vi "Subpanel.vi"() -> ()   [LabVIEW 2013]
panel:
  in  "Stop":bool
  in  "error in (no error)":errorcluster
  in  "RESET":bool
  in  "Feed Sel":bool
  in  "PCV Sel":bool
  in  "Boolean 10":bool
  in  "Boolean 9":bool
  in  "VLS Sel 1":bool
  in  "VLS Sel":bool
  in  "AKO Sel 2":bool
  in  "AKO Sel 1":bool
  in  "AKO Sel":bool
  in  "RX Sel":bool
  in  "MFC Sel":bool
  in  "Display Window":u16(ring) items=["Rx", "Guage", "PIDs", "Feed", "MFC", "AKO", "Steam", "Quench", "Back Half", "Heat Tapes"]
  in  "E-STOP":bool
  out "Estop":bool
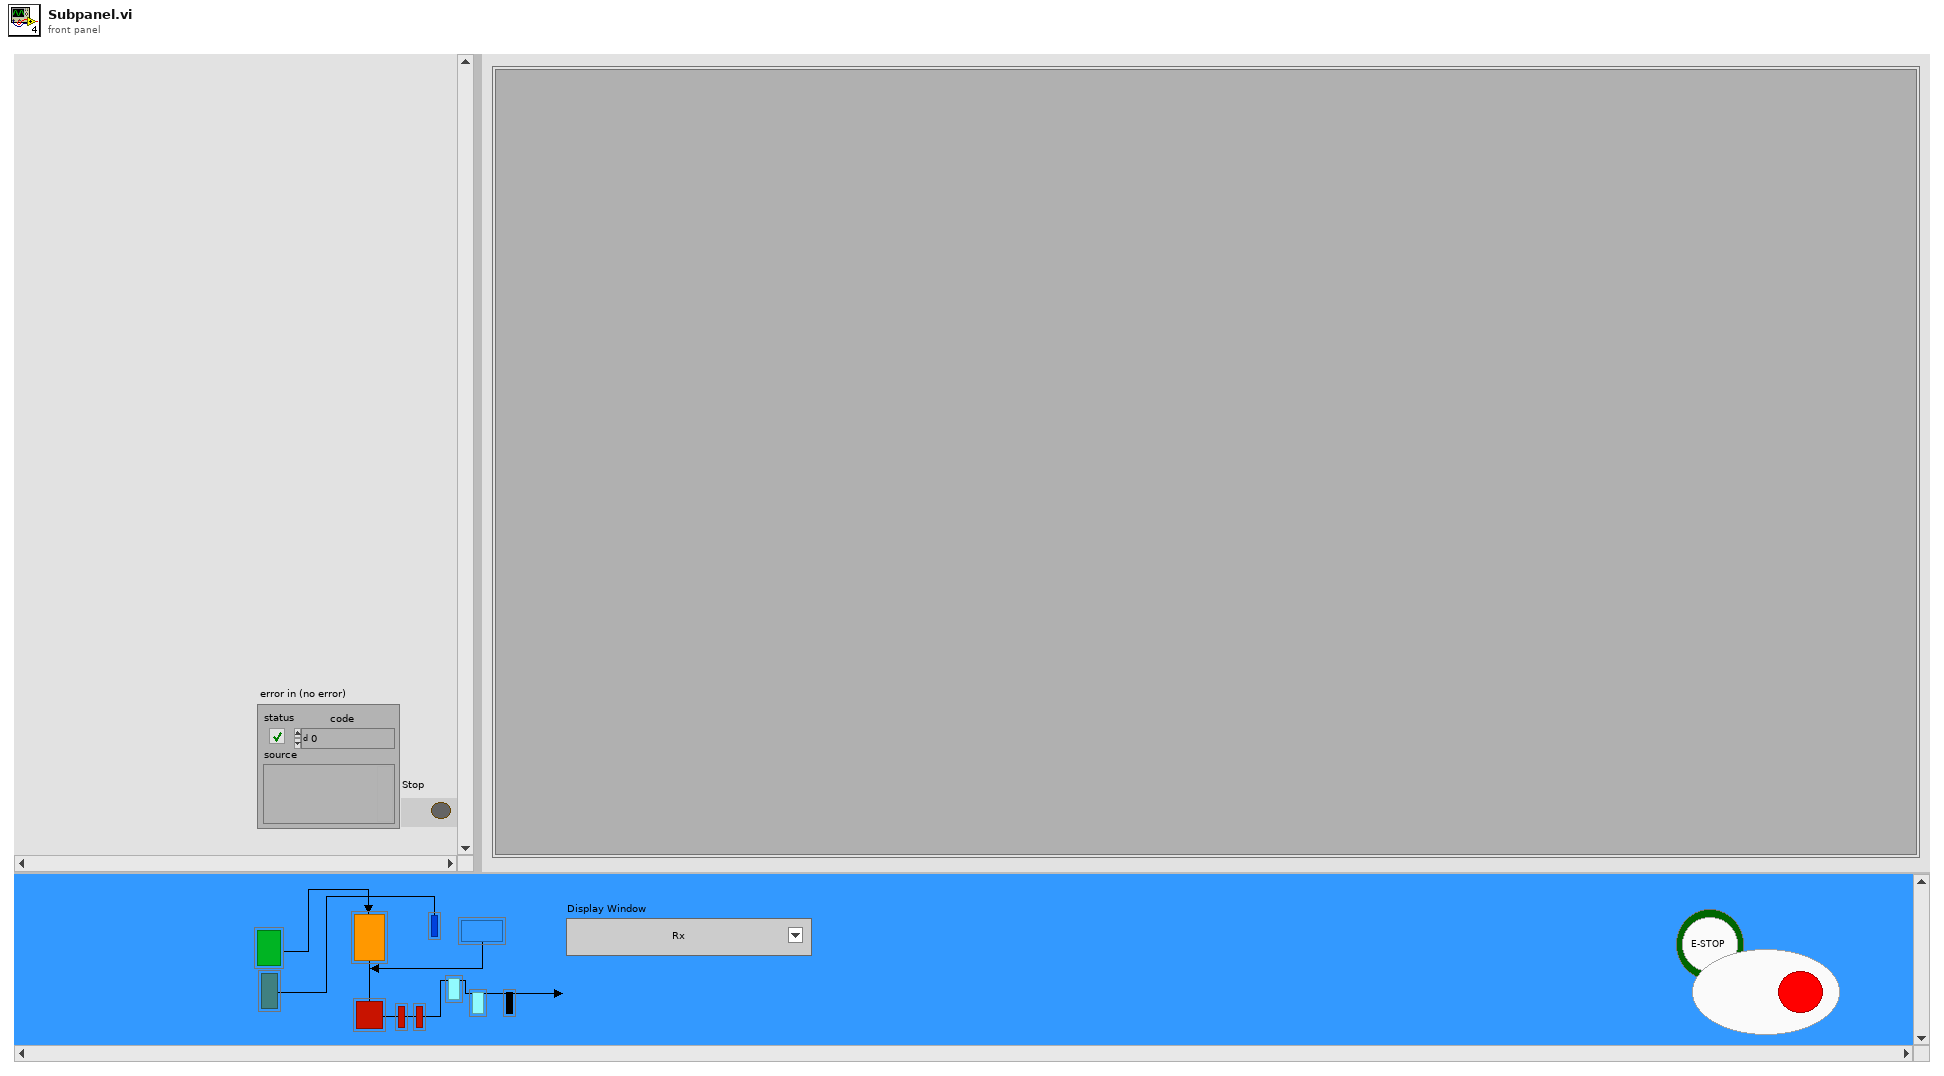
[diagram p1: front panel]
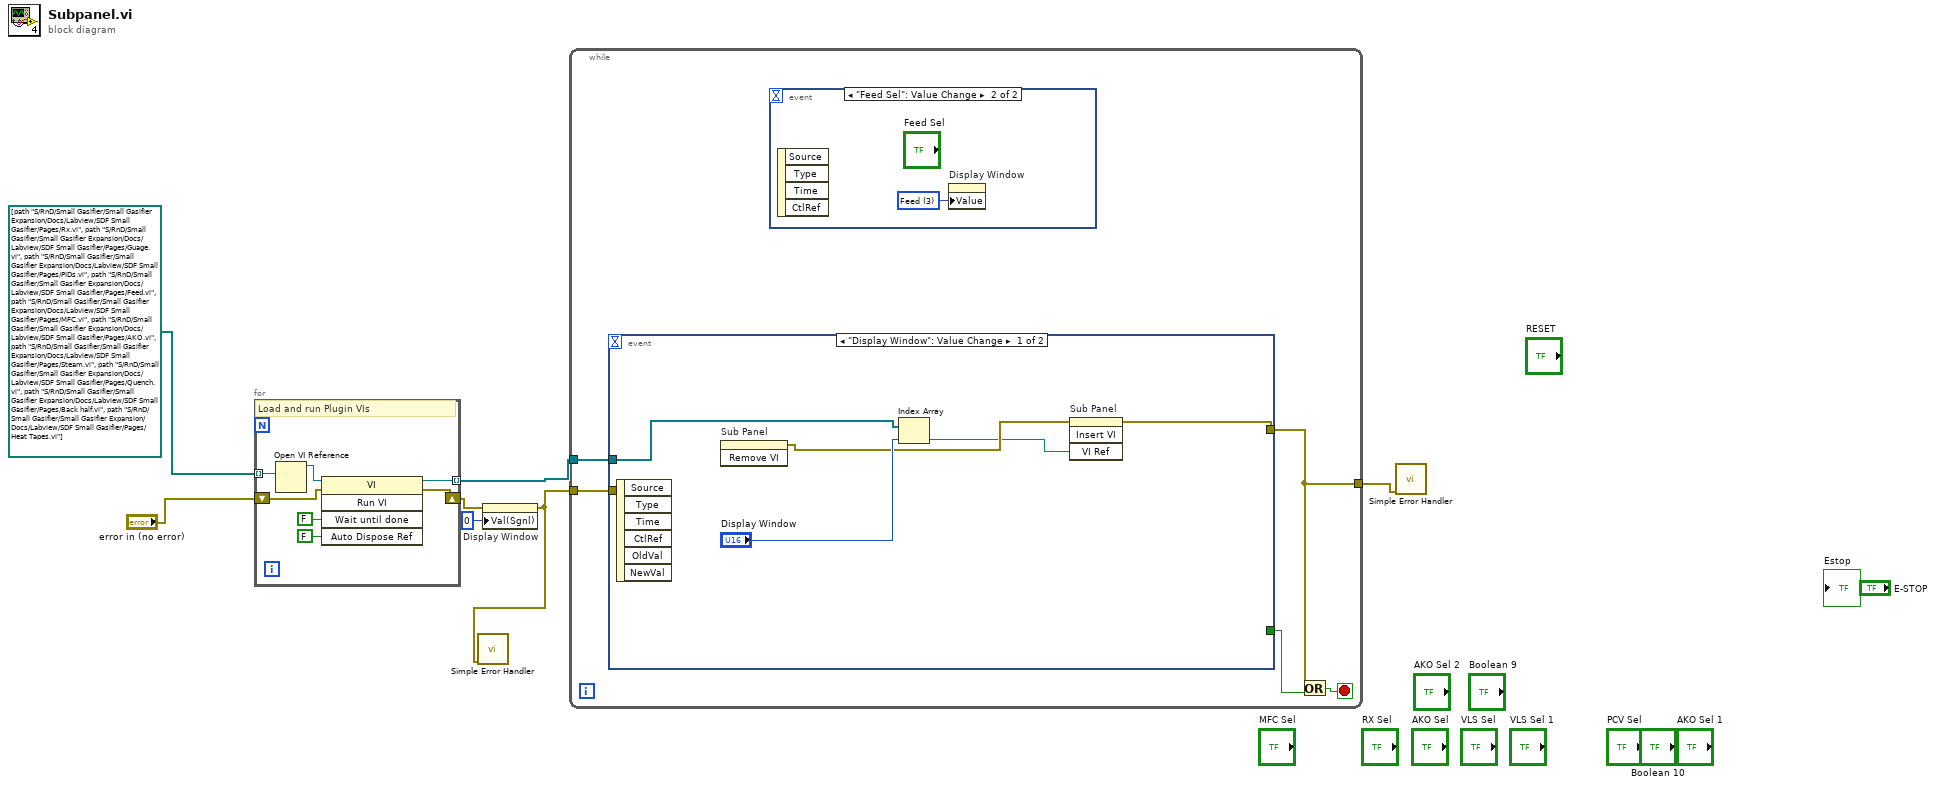
[diagram p0: block diagram]
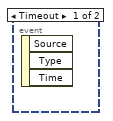
[diagram p2: hidden frame]
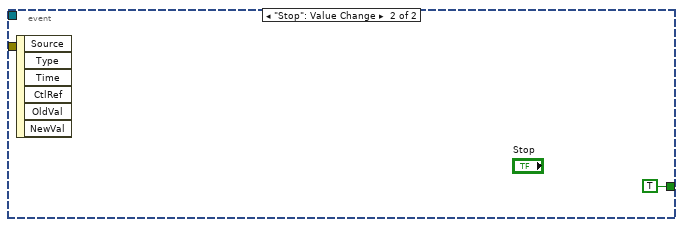
[diagram p3: hidden frame]
diagram:
  n1 = for {
    tunnel: [w13] -> w7 mode=indexing
    shift-right: [w12] -> w4
    shift-left: "error in (no error)" -> [w9]
    tunnel: path[] [path "S:/RnD/Small Gasifier/Small Gasifier Expansion/Docs/Labview/SDF Small Gasifier/Pages/Rx.vi", path "S:/RnD/Small Gasifier/Small Gasifier Expansion/Docs/Labview/SDF Small Gasifier/Pages/Guage.vi", path "S:/RnD/Small Gasifier/Small Gasifier Expansion/Docs/Labview/SDF Small Gasifier/Pages/PIDs.vi", path "S:/RnD/Small Gasifier/Small Gasifier Expansion/Docs/Labview/SDF Small Gasifier/Pages/Feed.vi", path "S:/RnD/Small Gasifier/Small Gasifier Expansion/Docs/Labview/SDF Small Gasifier/Pages/MFC.vi", path "S:/RnD/Small Gasifier/Small Gasifier Expansion/Docs/Labview/SDF Small Gasifier/Pages/AKO.vi", path "S:/RnD/Small Gasifier/Small Gasifier Expansion/Docs/Labview/SDF Small Gasifier/Pages/Steam.vi", path "S:/RnD/Small Gasifier/Small Gasifier Expansion/Docs/Labview/SDF Small Gasifier/Pages/Quench.vi", path "S:/RnD/Small Gasifier/Small Gasifier Expansion/Docs/Labview/SDF Small Gasifier/Pages/Back half.vi", path "S:/RnD/Small Gasifier/Small Gasifier Expansion/Docs/Labview/SDF Small Gasifier/Pages/Heat Tapes.vi"] -> [w8] mode=indexing
    # "Load and run Plugin VIs"
    n2 = Open VI Reference(vi path=w8) -> (vi reference=w14:refnum<vi>)  [unwired: 5 in, 1 out]
    n3 = invoke class="VI" method="Run VI"(reference=w14, error in=w9, "Wait until done"=FALSE ("Wait Until Done"), "Auto Dispose Ref"=FALSE ("Auto Dispose Reference")) -> (reference out=w13:refnum<vi>, error out=w12:errorcluster)  [unwired: 1 in, 3 out]
  }
  n4 = property on="Display Window" class="Ring (strict)"(error in=w4, "Val(Sgnl)"=u16 0 ("Value (Signaling)")) -> (error out=w2:errorcluster)  [unwired: 1 in, 1 out]
  n5 = call <vilib>:"Simple Error Handler.vi"("error in (no error)"=w2) -> ()  [unwired: 4 in, 5 out]
  n6 = while {
    tunnel: w7 -> [w19]
    tunnel: w2 -> [w18]
    tunnel: [w15] -> w5
    stop <- w17 stop-if-true
    n7 = event shown="[0] \"Display Window\": Value Change" {
      selector: _ -> [_ _]
      dyn-events: _ -> [_ _]
      timeout: _ -> [_ _]
      tunnel: w19 -> [w23 _]
      tunnel: w18 -> [_ _]
      tunnel: [w21 _] -> w15
      tunnel: [_ TRUE ("stop")] -> w16
      event "Display Window": Value Change {
        n8 = event-data() -> ()  [unwired: 1 in, 6 out]
        n9 = invoke on="Sub Panel" class="SubPnl" method="Remove VI"() -> (error out=w24:errorcluster)  [unwired: 3 in, 2 out]
        n10 = Index Array(array=w23, index="Display Window") -> (element=w22:refnum<vi>)
        n11 = invoke on="Sub Panel" class="SubPnl" method="Insert VI"(error in=w24, "VI Ref"=w22) -> (error out=w21:errorcluster)  [unwired: 2 in, 3 out]
      }
      event "Stop": Value Change {
        n12 = event-data() -> ()  [unwired: 1 in, 6 out]
      }
    }
    n13 = event shown="[1] \"Feed Sel\": Value Change" {
      selector: _ -> [_ _]
      dyn-events: _ -> [_ _]
      timeout: _ -> [_ _]
      event Timeout {
        n14 = event-data() -> ()  [unwired: 1 in, 3 out]
      }
      event "Feed Sel": Value Change {
        w20 = u16 3 items=["Rx", "Guage", "PIDs", "Feed", "MFC", "AKO", "Steam", "Quench", "Back Half", "Heat Tapes"] ("Display Window")
        n15 = event-data() -> ()  [unwired: 1 in, 4 out]
        n16 = property on="Display Window" class="Ring (strict)"("Value"=w20) -> ()  [unwired: 2 in, 2 out]
      }
    }
    n17 = Or(x=w15, y=w16) -> (x .or. y?=w17:bool)
  }
  n18 = call <vilib>:"Simple Error Handler.vi"("error in (no error)"=w5) -> ()  [unwired: 4 in, 5 out]
